vi "GOOP_GetOverrideMethods.vi"(1 "LvClassItem":refnum<vi>, 5 "error in (no error)":errorcluster) -> (15 "DynamicMethods(Names)":string[](array[string]), 16 "DynamicMehods(Paths)":path[](array[path]), 17 "Scope":T1(array[ring]), 18 "ConnectorPaneHeight":i32[](array[numeric]), 19 "error out":errorcluster)   [LabVIEW 2012]
panel:
  # "0 or -1 means Full Icon height\n1 is only one connector terminal height\n  and the header is then removed."
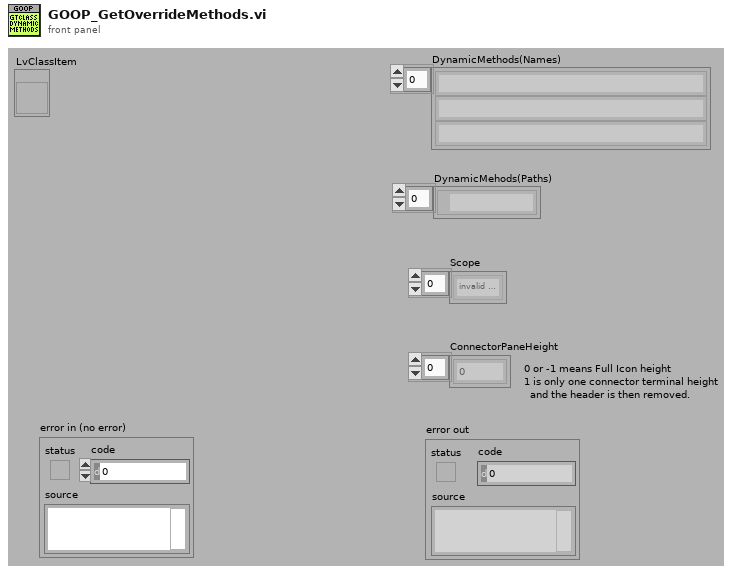
[diagram p1: front panel]
types:
  T1 = enum32{"invalid scope", "public", "private", "protected", "community"}[]
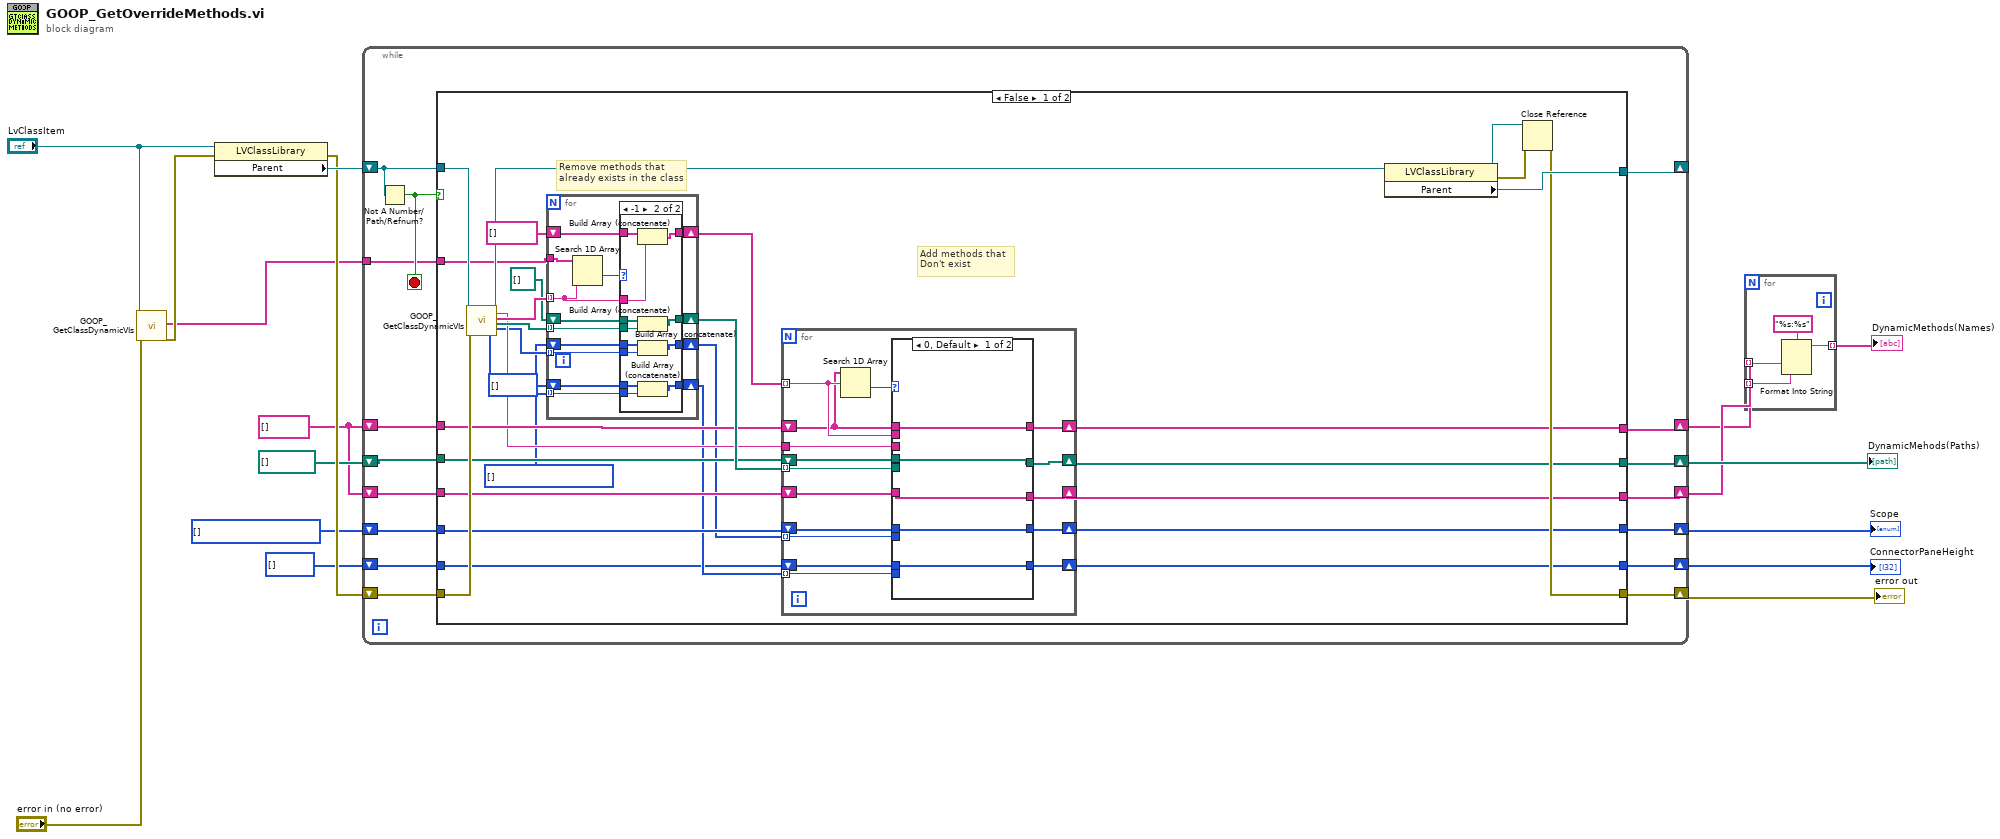
[diagram p0: block diagram]
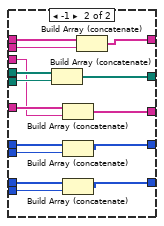
[diagram p3: hidden frame]
diagram:
  w4 = T1 [] items=["invalid scope", "public", "private", "protected", "community"]
  w9 = string[] []
  n1 = call <resource>:"GOOP_GetClassDynamicVIs.vi"("LvClassIn"="LvClassItem", "error out 2"="error in (no error)") -> ("VINames(without Prefix)"=w12:string[], "error out"=w13:errorcluster)  [unwired: 11 in, 5 out]
  n2 = property class="LVClassLibrary"(reference="LvClassItem", error in=w13) -> (error out=w16:errorcluster, "Parent"=w17:refnum<vi>)  [unwired: 1 out]
  n3 = while {
    shift-right: [w31] -> _
    shift-left: w17 -> [w32]
    shift-right: [w30] -> w15
    shift-left: w16 -> [w29]
    shift-right: [w27] -> w7
    shift-left: w9 -> [w28]
    tunnel: w12 -> [w26]
    shift-right: [w24] -> w11
    shift-left: path[] [] -> [w25]
    shift-right: [w22] -> w8
    shift-left: w9 -> [w23]
    shift-right: [w20] -> w3
    shift-left: w4 -> [w21]
    shift-right: [w19] -> w1
    shift-left: i32[] [] -> [w18]
    stop <- w33 stop-if-true
    n4 = Not A Number/Path/Refnum?(number/path/refnum=w32) -> (NaN/Path/Refnum?=w33:bool)
    n5 = case shown="False" w33 {
      tunnel: w32 -> [w59 w137]
      tunnel: [w64 w137] -> w31
      tunnel: [w61 w136] -> w30
      tunnel: w29 -> [w60 w136]
      tunnel: w28 -> [w51 w135]
      tunnel: [w50 w135] -> w27
      tunnel: w26 -> [w57 _]
      tunnel: w25 -> [w49 w134]
      tunnel: [w48 w134] -> w24
      tunnel: w23 -> [w46 w133]
      tunnel: [w45 w133] -> w22
      tunnel: w21 -> [w41 w132]
      tunnel: [w39 w132] -> w20
      tunnel: [w35 w131] -> w19
      tunnel: w18 -> [w34 w131]
      frame False {
        w42 = T1 [] items=["invalid scope", "public", "private", "protected", "community"]
        # "Add methods that\nDon't exist"
        # "Remove methods that\nalready exists in the class"
        n6 = call <resource>:"GOOP_GetClassDynamicVIs.vi"("LvClassIn"=w59, "error out 2"=w60) -> ("ConnectorPaneHeight"=w38:i32[], "LvClassOut"=w58:refnum<vi>, "ClassName"=w47:string, "VINames(without Prefix)"=w56:string[], "ViPaths"=w53:path[], "Scope"=w43:T1)  [unwired: 11 in, 1 out]
        n7 = for {
          tunnel: w57 -> [w78]
          tunnel: w56 -> [w74] mode=indexing
          shift-right: [w75] -> w54
          shift-left: string[] [] -> [w76]
          shift-right: [w71] -> w52
          shift-left: path[] [] -> [w73]
          tunnel: w53 -> [w72] mode=indexing
          shift-right: [w68] -> w40
          shift-left: w42 -> [w70]
          tunnel: w43 -> [w69] mode=indexing
          shift-right: [w67] -> w36
          shift-left: i32[] [] -> [w65]
          tunnel: w38 -> [w66] mode=indexing
          n8 = Search 1D Array(1D array=w78, element=w74) -> (index of element=w77:i32)  [unwired: 1 in]
          n9 = case shown="-1" w77 {
            tunnel: w76 -> [w82 w94]
            tunnel: [w82 w93] -> w75
            tunnel: w74 -> [_ w92]
            tunnel: w73 -> [w81 w91]
            tunnel: w72 -> [_ w90]
            tunnel: [w81 w89] -> w71
            tunnel: w70 -> [w80 w88]
            tunnel: w69 -> [_ w87]
            tunnel: [w80 w86] -> w68
            tunnel: w65 -> [w79 w83]
            tunnel: w66 -> [_ w84]
            tunnel: [w79 w85] -> w67
            frame 0, Default {
            }
            frame -1 {
              n10 = Build Array (concatenate)(w94, w92) -> (w93:string[])
              n11 = Build Array (concatenate)(w91, w90) -> (w89:path[])
              n12 = Build Array (concatenate)(w88, w87) -> (w86:T1)
              n13 = Build Array (concatenate)(w83, w84) -> (w85:i32[])
            }
          }
        }
        n14 = for {
          tunnel: w54 -> [w109] mode=indexing
          tunnel: w52 -> [w108] mode=indexing
          shift-right: [w106] -> w50
          shift-left: w51 -> [w107]
          shift-right: [w104] -> w48
          shift-left: w49 -> [w105]
          tunnel: w47 -> [w103]
          shift-right: [w101] -> w45
          shift-left: w46 -> [w102]
          shift-right: [w98] -> w39
          shift-left: w41 -> [w100]
          tunnel: w40 -> [w99] mode=indexing
          shift-right: [w97] -> w35
          shift-left: w34 -> [w95]
          tunnel: w36 -> [w96] mode=indexing
          n15 = Search 1D Array(1D array=w107, element=w109) -> (index of element=w110:i32)  [unwired: 1 in]
          n16 = case shown="0, Default" w110 {
            tunnel: w107 -> [w115 w130]
            tunnel: [w115 w129] -> w106
            tunnel: w109 -> [_ w123]
            tunnel: w108 -> [_ w128]
            tunnel: w105 -> [w114 w127]
            tunnel: [w114 w126] -> w104
            tunnel: w103 -> [_ w124]
            tunnel: w102 -> [w113 w125]
            tunnel: [w113 w122] -> w101
            tunnel: w100 -> [w112 w121]
            tunnel: w99 -> [_ w120]
            tunnel: [w112 w119] -> w98
            tunnel: w95 -> [w111 w116]
            tunnel: w96 -> [_ w117]
            tunnel: [w111 w118] -> w97
            frame 0, Default {
            }
            frame -1 {
              n17 = Build Array (concatenate)(w127, w128) -> (w126:path[])
              n18 = Build Array (concatenate)(w125, w124) -> (w122:string[])
              n19 = Build Array (concatenate)(w121, w120) -> (w119:T1)
              n20 = Build Array (concatenate)(w116, w117) -> (w118:i32[])
              n21 = Build Array (concatenate)(w130, w123) -> (w129:string[])
            }
          }
        }
        n22 = property class="LVClassLibrary"(reference=w58) -> (reference out=w62:refnum<vi>, error out=w63:errorcluster, "Parent"=w64:refnum<vi>)  [unwired: 1 in]
        n23 = Close Reference(reference=w62, error in (no error)=w63) -> (error out=w61:errorcluster)
      }
      frame True {
      }
    }
  }
  "error out" <- w15
  "DynamicMehods(Paths)" <- w11
  "Scope" <- w3
  "ConnectorPaneHeight" <- w1
  n24 = for {
    tunnel: w8 -> [w140] mode=indexing
    tunnel: w7 -> [w139] mode=indexing
    tunnel: [w138] -> w6 mode=indexing
    n25 = Format Into String(format string="%s:%s", w140, w139) -> (resulting string=w138:string)  [unwired: 2 in, 1 out]
  }
  "DynamicMethods(Names)" <- w6
